vi "API Cache.vi"(8 "error in":errorcluster, 9 "Action":enum16{"Initialize", "Get or Open", "Clear"}(ring), 11 "VI Path":path) -> (0 "error out":errorcluster, 3 "VI Reference":refnum<vi>)   [LabVIEW 2021, in "Acquisition.lvlib"]
uses:
  Acquisition.lvlib
  f30a3141-783f-4f77-96a1-60bf18835bb9.vi
panel:
  out "Cache":map{path, refnum<vi>}(c390)
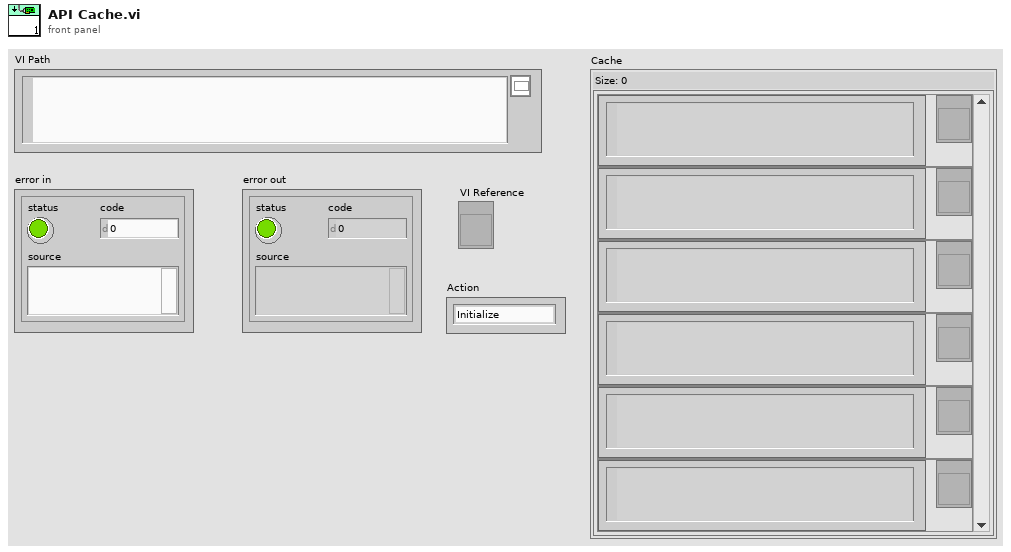
[diagram p1: front panel]
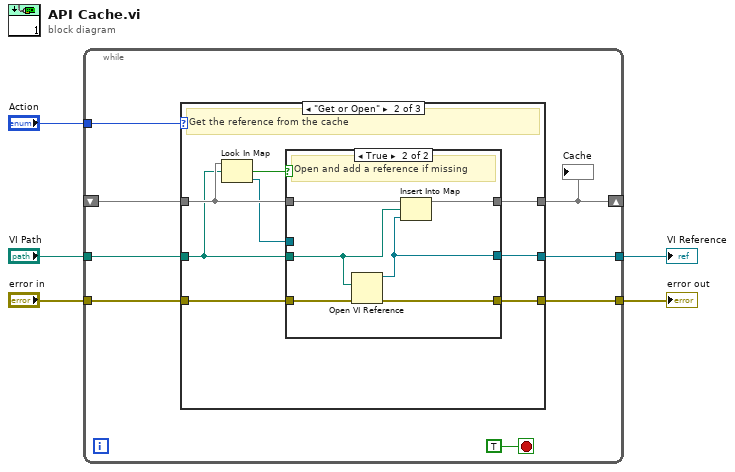
[diagram p0: block diagram]
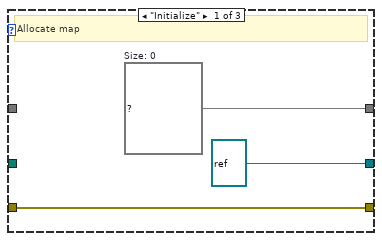
[diagram p2: hidden frame]
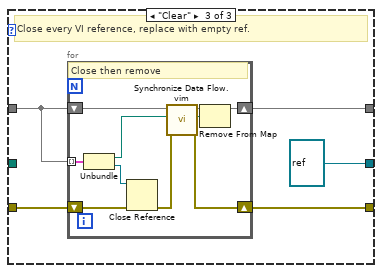
[diagram p4: hidden frame]
diagram:
  n1 = while {
    shift-right: [w12] -> _
    shift-left: _ -> [w11]
    tunnel: "VI Path" -> [w10]
    tunnel: [w9] -> w4
    tunnel: "error in" -> [w8]
    tunnel: [w7] -> w2
    tunnel: "Action" -> [w6]
    stop <- TRUE stop-if-true
    n2 = case shown="\"Get or Open\"" w6 {
      tunnel: [w16 w24 w36] -> w12
      tunnel: w11 -> [_ w23 w37]
      tunnel: w10 -> [_ w21 _]
      tunnel: [refnum<vi> refnum ("vi reference") w20 refnum<vi> refnum ("vi reference")] -> w9
      tunnel: w8 -> [w14 w19 w38]
      tunnel: [w14 w18 w35] -> w7
      frame "Initialize" {
        w16 = map{path, refnum<vi>} {}  # Size: 0
        # "Allocate map"
      }
      frame "Get or Open" {
        # "Get the reference from the cache"
        n3 = Look In Map(map=w23, key=w21) -> (key not found?=w22:bool, value=w17:refnum<vi>)  [unwired: 1 in]
        n4 = case shown="True" w22 {
          tunnel: [w25 w33] -> w24
          tunnel: w23 -> [w25 w32]
          tunnel: w21 -> [_ w28]
          tunnel: w19 -> [w26 w31]
          tunnel: [w26 w30] -> w18
          tunnel: [w27 w29] -> w20
          tunnel: w17 -> [w27 _]
          frame False {
          }
          frame True {
            # "Open and add a reference if missing"
            n5 = Open VI Reference(vi path=w28, error in (no error)=w31) -> (vi reference=w29:refnum<vi>, error out=w30:errorcluster)  [unwired: 4 in]
            n6 = Insert Into Map(map in=w32, key=w28, value=w29) -> (map out=w33:map{path, refnum<vi>})  [unwired: 2 out]
          }
        }
      }
      frame "Clear" {
        # "Close every VI reference, replace with empty ref."
        n7 = for {
          tunnel: w37 -> [w46] mode=indexing
          shift-right: [w39] -> w35
          shift-left: w38 -> [w48]
          shift-right: [w45] -> w36
          shift-left: w37 -> [w44]
          # "Close then remove"
          n8 = Unbundle(w46) -> ("VI Path"=w43:path, "VI Reference"=w47:refnum<vi>)
          n9 = Close Reference(reference=w47, error in (no error)=w48) -> (error out=w40:errorcluster)
          n10 = call "Synchronize Data Flow.vim"("input 4"=w40, "input 2"=w43, "input 1"=w44) -> ("output 4"=w39:errorcluster, "output 2"=w41:path, "output 1"=w42:map{path, refnum<vi>})  [unwired: 1 in, 1 out]
          n11 = Remove From Map(10:w41, 11:w42) -> (3:w45:map{path, refnum<vi>})  [unwired: 2 out]
        }
      }
    }
    "Cache" <- w12
  }
  "VI Reference" <- w4
  "error out" <- w2
